vi "Delete Me.vi"() -> ()   [LabVIEW 2019, in "36234A.lvlib" / "36234A.lvclass"]
uses:
  Library/36234A.lvclass
  C:/Users/Public/Documents/Development/builds/Instruments/Instruments.lvlibp/Library/Instruments.lvclass
  builds/Instruments/Instruments.lvlibp/Accessors/Write Resource.vi
panel:
  in  "byte count":u32=512
  in  "Reset":bool
  out "RESPONSE":string
  in  "Query":bool
  in  "Command":bool
  in  "CMD":string
  in  "stop":bool
  out "error out":errorcluster
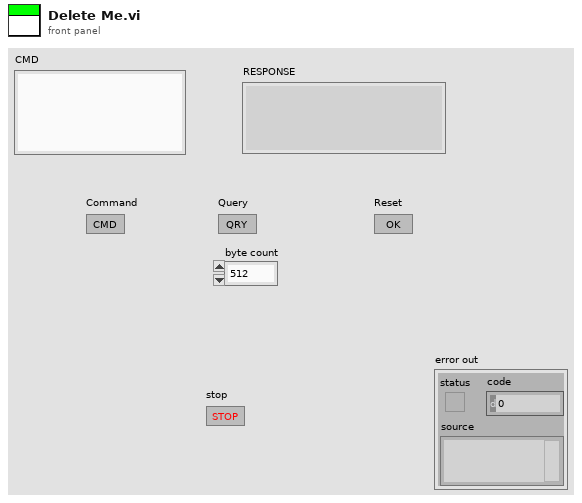
[diagram p1: front panel]
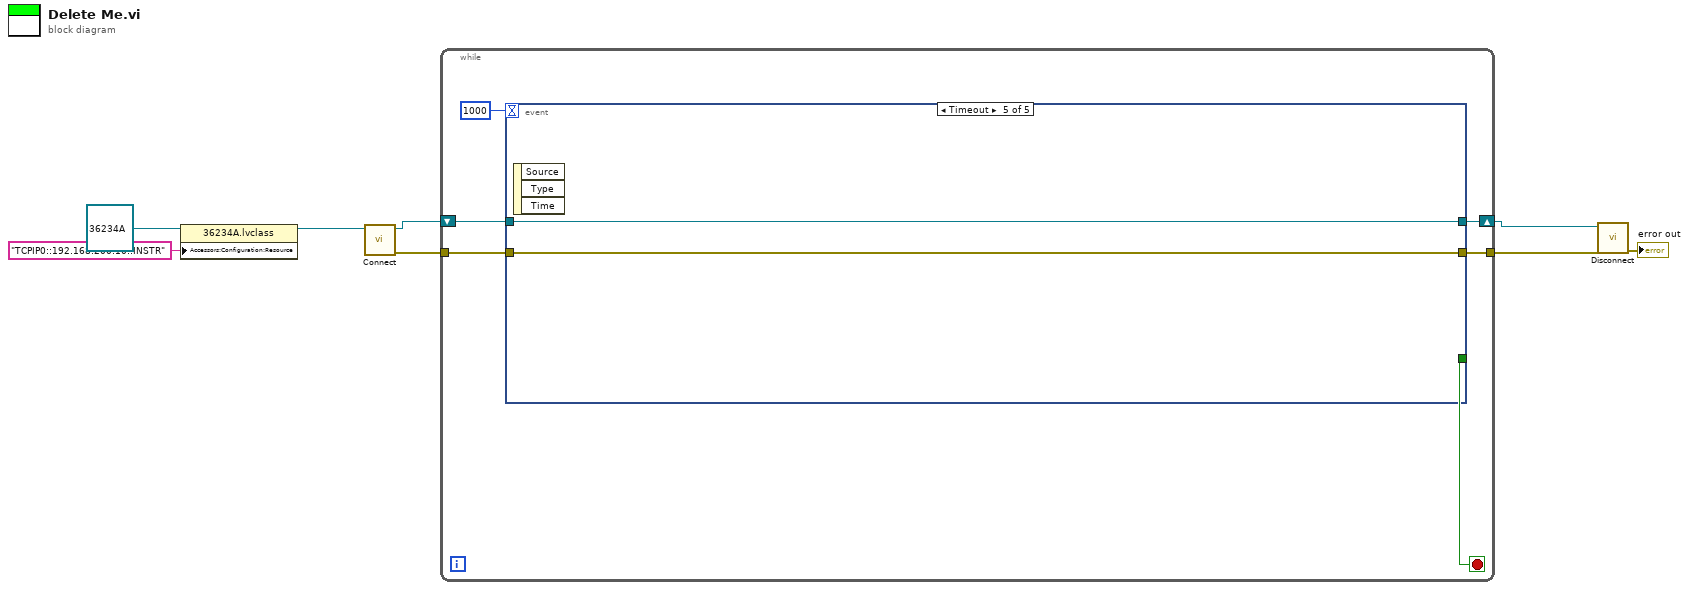
[diagram p0: block diagram]
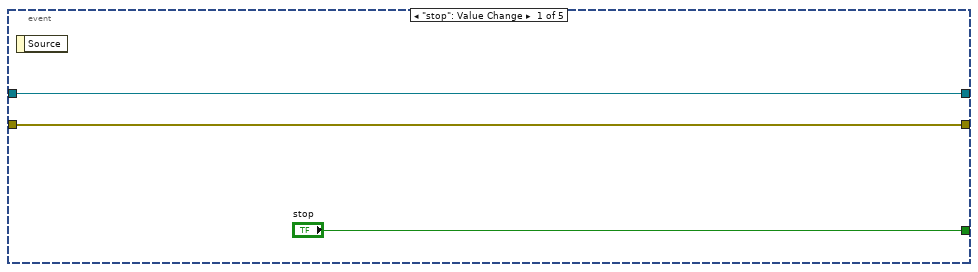
[diagram p2: hidden frame]
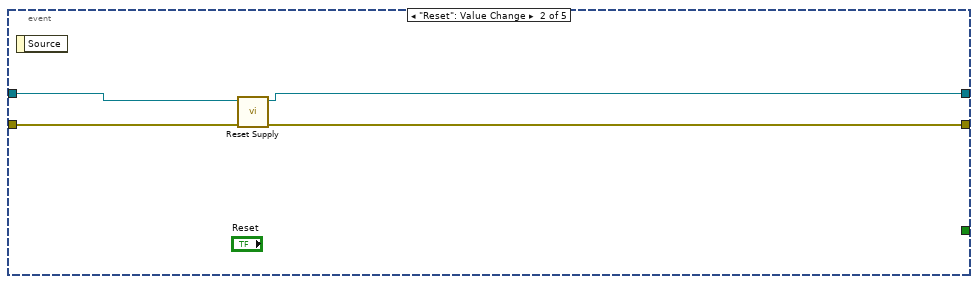
[diagram p3: hidden frame]
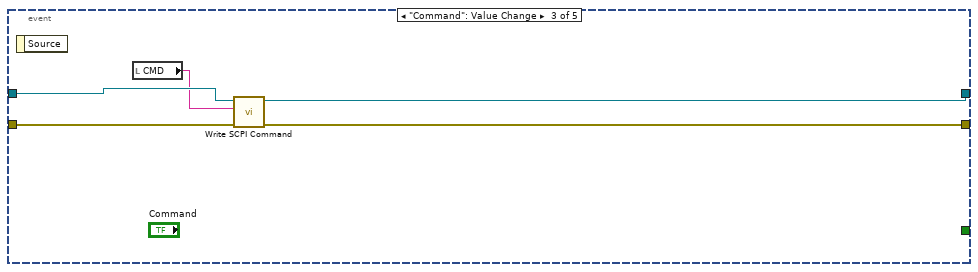
[diagram p4: hidden frame]
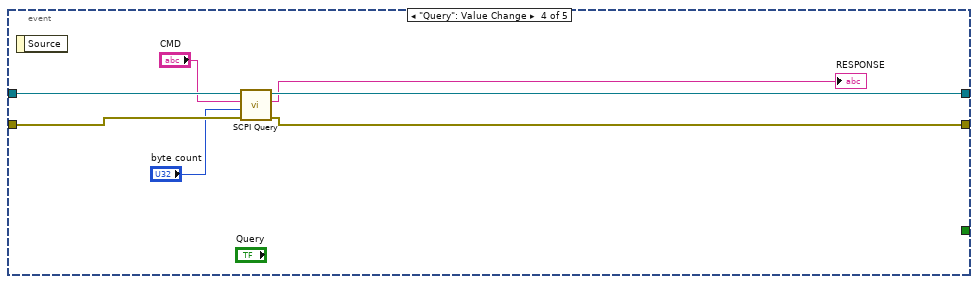
[diagram p5: hidden frame]
diagram:
  n1 = property class="36234A.lvclass"(reference=refnum<class "36234A.lvclass"> refnum ("36234A.lvlib:36234A.lvclass"), "Accessors:Configuration:Resource"="TCPIP0::192.168.200.10::INSTR" ("Instrument:Config:Resource")) -> (reference out=w6:refnum<class "36234A.lvclass">)  [unwired: 1 in, 1 out]
  n2 = call-dynamic "Connect.vi"("36234A in"=w6) -> ("error out"=w2:errorcluster, "36234A out"=w4:refnum<class "36234A.lvclass">)  [unwired: 9 in]
  n3 = while {
    shift-right: [w12] -> w3
    shift-left: w4 -> [w13]
    tunnel: w2 -> [w11]
    tunnel: [w10] -> w1
    stop <- w14 stop-if-true
    n4 = event shown="[4] Timeout" {
      selector: _ -> [_ _ _ _ _]
      dyn-events: _ -> [_ _ _ _ _]
      timeout: 1000 -> [_ _ _ _ _]
      tunnel: ["stop" _ _ _ _] -> w14
      tunnel: w13 -> [w16 w19 w26 w33 w35]
      tunnel: [w16 w18 w24 w31 w35] -> w12
      tunnel: w11 -> [w15 w21 w25 w32 w34]
      tunnel: [w15 w20 w23 w30 w34] -> w10
      event "stop": Value Change {
        n5 = event-data() -> ()  [unwired: 1 in, 1 out]
      }
      event "Reset": Value Change {
        n6 = event-data() -> ()  [unwired: 1 in, 1 out]
        n7 = call-dynamic "Reset Supply.vi"("error in"=w21, "36234A in"=w19) -> ("error out"=w20:errorcluster, "36234A out"=w18:refnum<class "36234A.lvclass">)  [unwired: 8 in]
      }
      event "Command": Value Change {
        n8 = event-data() -> ()  [unwired: 1 in, 1 out]
        n9 = local read "CMD"() -> (w22:string)
        n10 = call "Write SCPI Command.vi"("error in (no error)"=w25, "SCPI Command"=w22, "36234A in"=w26) -> ("error out"=w23:errorcluster, "36234A out"=w24:refnum<class "36234A.lvclass">)  [unwired: 7 in]
      }
      event "Query": Value Change {
        n11 = event-data() -> ()  [unwired: 1 in, 1 out]
        n12 = call "SCPI Query.vi"("error in (no error)"=w32, "byte count"="byte count", "SCPI QUERY"="CMD", "36234A in"=w33) -> ("error out"=w30:errorcluster, "read buffer"=→"RESPONSE":string, "36234A out"=w31:refnum<class "36234A.lvclass">)  [unwired: 5 in]
      }
      event Timeout {
        n13 = event-data() -> ()  [unwired: 1 in, 3 out]
      }
    }
  }
  n14 = call-dynamic "Disconnect.vi"("error in"=w1, "36234A in"=w3) -> ("error out"=→"error out":errorcluster)  [unwired: 8 in, 1 out]
